vi "test Description.vi"(8 "error in (no error)":errorcluster, 11 "TestCase in":refnum<class "Parameter Setting.lvclass">) -> (0 "error out":errorcluster, 3 "TestCase out":refnum<class "Parameter Setting.lvclass">)   [LabVIEW 2017, in "Deterministic Error Tests.lvlib" / "Parameter Setting.lvclass"]
uses:
  Parameter Setting.lvclass
  Parameter Setting.lvclass/Parameter Setting.ctl
  <vilib>/addons/_JKI Toolkits/VI Tester/TestCase.llb/TestCase.lvclass
  Source/Deterministic Error Builder.lvlib
  C:/Program Files (x86)/National Instruments/LabVIEW 2017/vi.lib/addons/_JKI Toolkits/VI Tester/TestCase.llb/TestCase.lvclass
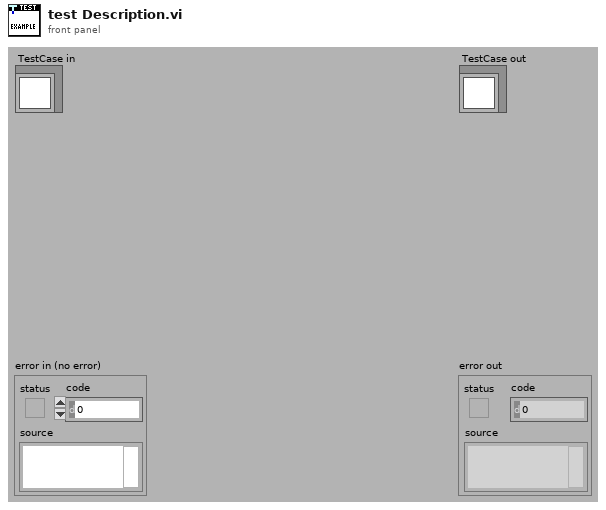
[diagram p1: front panel]
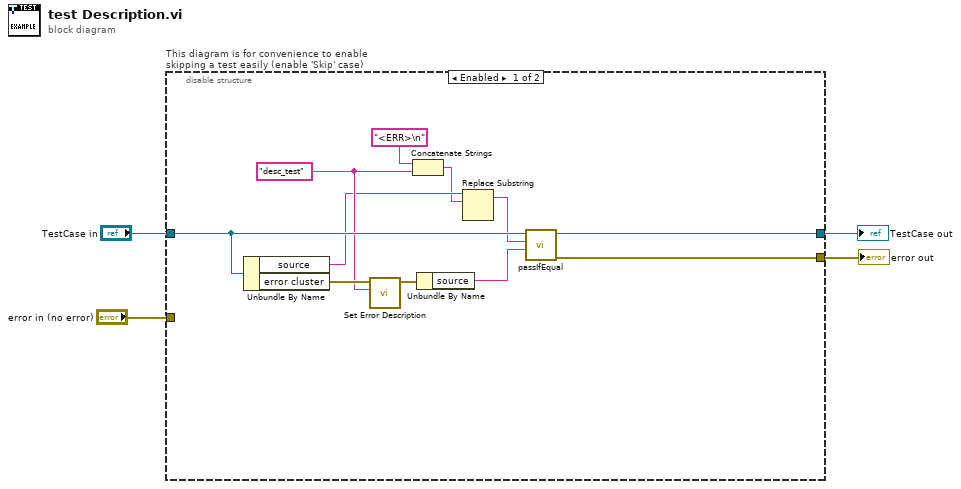
[diagram p0: block diagram]
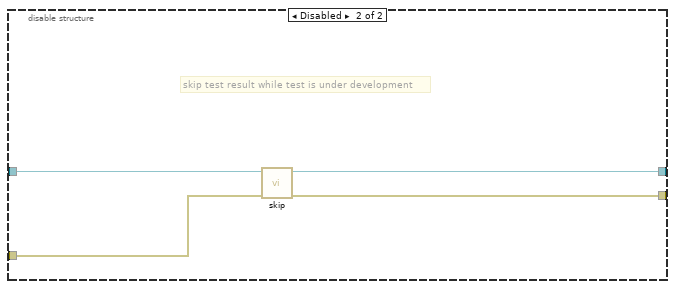
[diagram p2: hidden frame]
diagram:
  n1 = disable-structure "This diagram is for convenience to enable skipping a test easily (enable 'Skip' case)" shown="Enabled" {
    disable-tunnel: "TestCase in" -> [w14 w19]
    disable-tunnel: [w15 w17] -> w2
    disable-tunnel: [w8 w18] -> w1
    disable-tunnel: "error in (no error)" -> [_ w16]
    frame Enabled {
      w10 = "desc_test"
      n2 = Unbundle By Name(w14) -> ("source"=w9:string, "error cluster"=w13:errorcluster)
      n3 = call "Set Error Description.vi"("error description"=w10, "error in"=w13) -> ("error out"=w7:errorcluster)  [unwired: 8 in, 1 out]
      n4 = Concatenate Strings("<ERR>\n", w10) -> (w6:string)
      n5 = Unbundle By Name(w7) -> ("source"=w12:string)
      n6 = Replace Substring(4:w6, 5:w9) -> (1:w5:string)  [unwired: 2 in, 1 out]
      n7 = call-dynamic "passIfEqual.vi"("y"=w12, "x"=w5, "TestCase in"=w14) -> ("error out"=w8:errorcluster, "TestCase out"=w15:refnum<class "Parameter Setting.lvclass">)  [unwired: 7 in]
    }
    frame Disabled {
      # "skip test result while test is under development"
      n8 = call <vilib>:"skip.vi"("error in (no error)"=w16, "TestCase in"=w19) -> ("error out"=w18:errorcluster, "TestCase out"=w17:refnum<class "Parameter Setting.lvclass">)  [unwired: 8 in]
    }
  }
  "error out" <- w1
  "TestCase out" <- w2
